vi "Read Data Titles.vi"(8 "error in (no error)":errorcluster, 11 "EGG5302 in":refnum<class "EGG5302.lvclass">) -> (0 "error out":errorcluster, 2 "Data titles":string[](array[string])=["EGG5302_Vx (V)", "EGG5302_Vy (V)"], 3 "EGG5302 out":refnum<class "EGG5302.lvclass">)   [LabVIEW 2015, in "EGG5302.lvclass"]
uses:
  EGG5302.lvclass
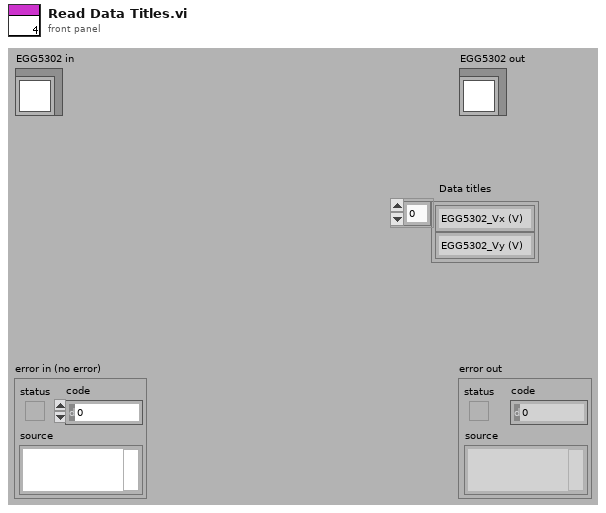
[diagram p1: front panel]
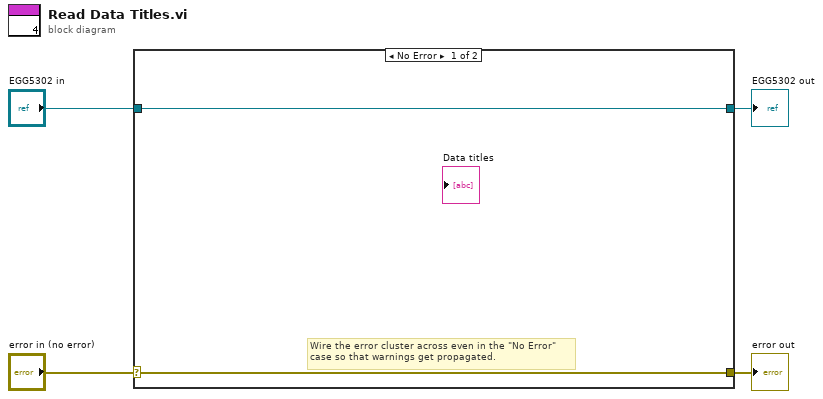
[diagram p0: block diagram]
diagram:
  n1 = case shown="No Error" "error in (no error)" {
    selector: "error in (no error)" -> [w5 w8]
    tunnel: [w5 w8] -> w3
    tunnel: [w6 w7] -> w1
    tunnel: "EGG5302 in" -> [w6 w7]
    frame No Error {
      # "Wire the error cluster across even in the \"No Error\"\ncase so that warnings get propagated."
    }
    frame Error {
    }
  }
  "error out" <- w3
  "EGG5302 out" <- w1
